vi "data preparer.vi"(2 "error in (no error)":errorcluster, 3 "UI Data":T2) -> (0 "error out":errorcluster, 1 "Prepared (Infix) Data":T1)   [LabVIEW 2020]
uses:
  controls/UI Data.ctl
  <vilib>/Utility/error.llb/Error Cluster From Error Code.vi
  <vilib>/ErrorRing/Error Ring.xnode
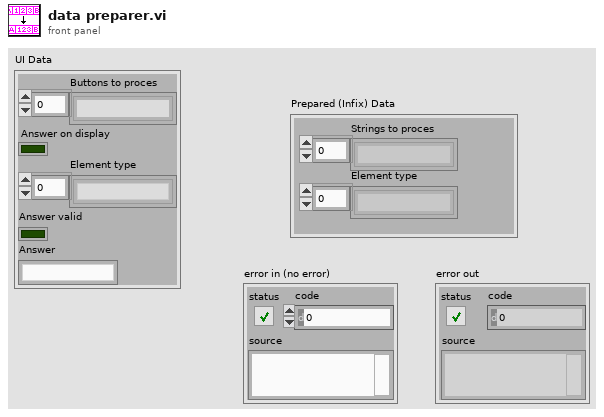
[diagram p1: front panel]
types:
  T1 = cluster{"Strings to proces":string[], "Element type":string[]}
  T2 = typedef "UI Data.ctl" = cluster{"Buttons to proces":string[], "Answer on display":bool, "Element type":string[], "Answer valid":bool, "Answer":string}
  T3 = cluster{"Buttons to proces":string[], "Element type":string[]}
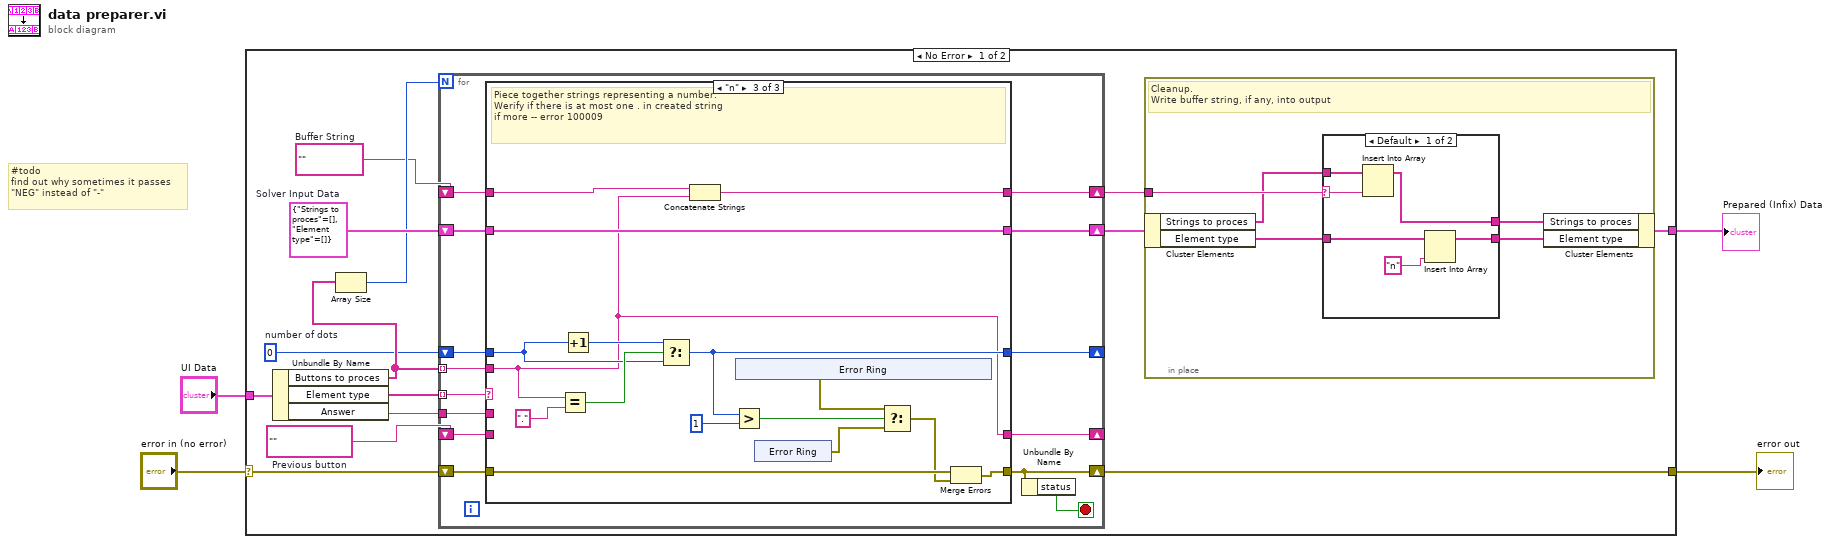
[diagram p0: block diagram]
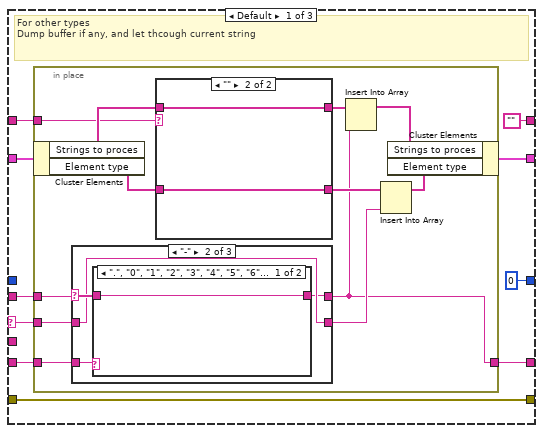
[diagram p3: hidden frame]
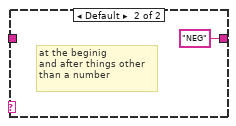
[diagram p5: hidden frame]
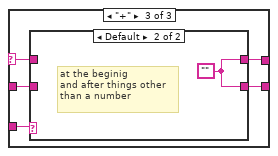
[diagram p6: hidden frame]
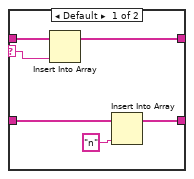
[diagram p8: hidden frame]
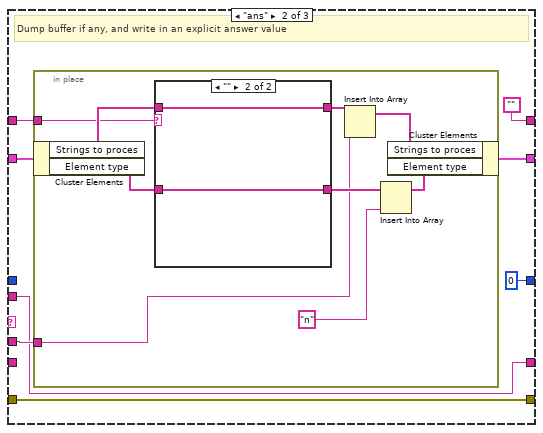
[diagram p9: hidden frame]
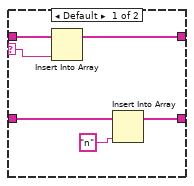
[diagram p10: hidden frame]
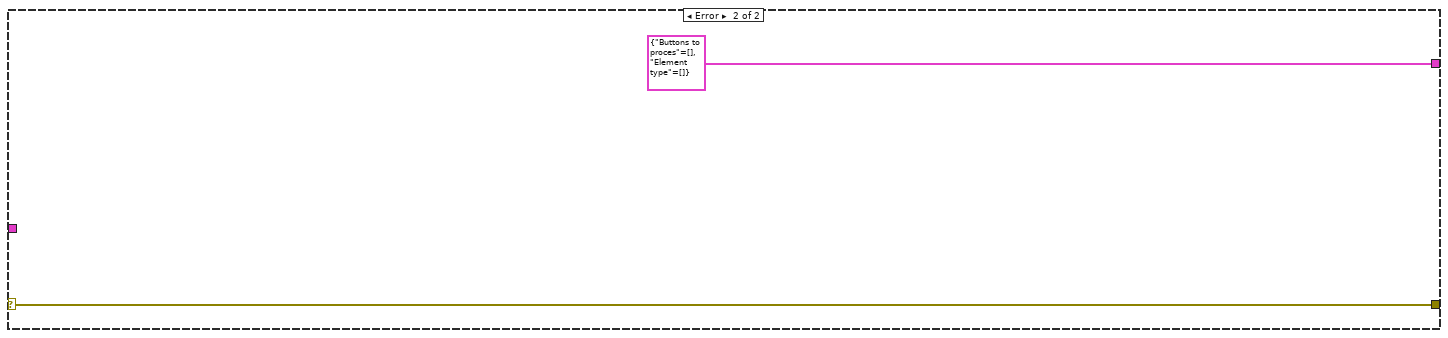
[diagram p11: hidden frame]
diagram:
  # "#todo\nfind out why sometimes it passes\n\"NEG\" instead of \"-\""
  n1 = case shown="No Error" "error in (no error)" {
    selector: "error in (no error)" -> [w16 w140]
    tunnel: [w10 w140] -> w3
    tunnel: "UI Data" -> [w17 _]
    tunnel: [w11 T3 {"Buttons to proces"=[], "Element type"=[]} ("Solver Input Data")] -> w1
    frame No Error {
      w5 = ""  # Previous button
      w6 = 0  # number of dots
      w14 = ""  # Buffer String
      w18 = T1 {"Strings to proces"=[], "Element type"=[]}  # Solver Input Data
      n2 = Unbundle By Name(w17) -> ("Buttons to proces"=w7:string[], "Element type"=w9:string[], "Answer"=w8:string)
      n3 = Array Size(array=w7) -> (size(s)=w15:i32)
      n4 = for {
        N: w15 -> [_]
        shift-right: [w44] -> w12
        shift-left: w18 -> [w45]
        shift-right: [w35] -> w10
        shift-left: w16 -> [w43]
        shift-right: [w41] -> w13
        shift-left: w14 -> [w42]
        tunnel: w7 -> [w40] mode=indexing
        tunnel: w9 -> [w39] mode=indexing
        tunnel: w8 -> [w38]
        shift-right: [w36] -> _
        shift-left: w6 -> [w37]
        shift-right: [w32] -> _
        shift-left: w5 -> [w33]
        stop <- w34 stop-if-true
        n5 = case shown="\"n\"" w39 {
          selector: w39 -> [w52 _ _]
          tunnel: w45 -> [w54 w98 w132]
          tunnel: [w53 w97 w132] -> w44
          tunnel: w43 -> [w55 w99 w131]
          tunnel: [w55 w99 w119] -> w35
          tunnel: w40 -> [w51 w92 w117]
          tunnel: w42 -> [w49 w95 w130]
          tunnel: ["" "" w129] -> w41
          tunnel: w38 -> [_ w94 _]
          tunnel: w37 -> [_ _ w125]
          tunnel: [0 ("number of dots") 0 ("number of dots") w124] -> w36
          tunnel: w33 -> [w47 _ _]
          tunnel: [w46 w92 w117] -> w32
          frame Default {
            # "For other types\nDump buffer if any, and let thcough current string"
            n6 = in-place {
              in-place-border: w52 -> [w60]
              in-place-border: w51 -> [w58]
              in-place-border: w49 -> [w61]
              in-place-border: w47 -> [w57]
              in-place-border: [w56] -> w46
              n7 = in-place-cluster #1(w54) -> ("Strings to proces"=w65:string[], "Element type"=w64:string[])
              n8 = case shown="\"-\"" w58 {
                selector: w58 -> [w68 w71 w79]
                tunnel: [w68 w70 w78] -> w56
                tunnel: w60 -> [w69 w72 w77]
                tunnel: [w69 w72 w76] -> w59
                tunnel: w57 -> [_ w73 w80]
                frame Default {
                  # "things other than \"-\" and \"+\""
                }
                frame "-" {
                  n9 = case shown="\".\", \"0\", \"1\", \"2\", \"3\", \"4\", \"5\", \"6\", \"7\", \"8\", \"9\", \"Ans\"" w73 {
                    tunnel: w71 -> [w74 _]
                    tunnel: [w74 "NEG"] -> w70
                    frame ".", "0", "1", "2", "3", "4", "5", "6", "7", "8", "9", "Ans" {
                    }
                    frame Default {
                      # "at the beginig\nand after things other \nthan a number"
                    }
                  }
                }
                frame "+" {
                  n10 = case shown="Default" w80 {
                    tunnel: w79 -> [w82 _]
                    tunnel: [w82 w83] -> w78
                    tunnel: w77 -> [w81 _]
                    tunnel: [w81 w83] -> w76
                    frame ".", "0", "1", "2", "3", "4", "5", "6", "7", "8", "9" {
                    }
                    frame Default {
                      w83 = ""
                      # "at the beginig\nand after things other \nthan a number"
                    }
                  }
                }
              }
              n11 = case shown="\"\"" w61 {
                selector: w61 -> [w85 _]
                tunnel: w65 -> [w89 w91]
                tunnel: [w88 w91] -> w62
                tunnel: w64 -> [w87 w90]
                tunnel: [w86 w90] -> w63
                frame Default {
                  n12 = Insert Into Array(array=w89, new element=w85) -> (w88:string[])  [unwired: 1 in]
                  n13 = Insert Into Array(array=w87, new element="n" ("new element/subarray")) -> (w86:string[])  [unwired: 1 in]
                }
                frame "" {
                }
              }
              n14 = Insert Into Array(array=w62, new element=w56) -> (w67:string[])  [unwired: 1 in]
              n15 = Insert Into Array(array=w63, new element=w59) -> (w66:string[])  [unwired: 1 in]
              n16 = in-place-cluster #1("Strings to proces"=w67, "Element type"=w66) -> (w53:T1)
            }
          }
          frame "ans" {
            # "Dump buffer if any, and write in an explicit answer value"
            n17 = in-place {
              in-place-border: w95 -> [w102]
              in-place-border: w94 -> [w100]
              n18 = in-place-cluster #2(w98) -> ("Strings to proces"=w106:string[], "Element type"=w105:string[])
              n19 = case shown="\"\"" w102 {
                selector: w102 -> [w110 _]
                tunnel: w106 -> [w114 w116]
                tunnel: [w113 w116] -> w103
                tunnel: w105 -> [w112 w115]
                tunnel: [w111 w115] -> w104
                frame Default {
                  n20 = Insert Into Array(array=w114, new element=w110) -> (w113:string[])  [unwired: 1 in]
                  n21 = Insert Into Array(array=w112, new element="n" ("new element/subarray")) -> (w111:string[])  [unwired: 1 in]
                }
                frame "" {
                }
              }
              n22 = Insert Into Array(array=w103, new element=w100) -> (w108:string[])  [unwired: 1 in]
              n23 = Insert Into Array(array=w104, new element="n") -> (w107:string[])  [unwired: 1 in]
              n24 = in-place-cluster #2("Strings to proces"=w108, "Element type"=w107) -> (w97:T1)
            }
          }
          frame "n" {
            # "Piece together strings representing a number.\nWerify if there is at most one . in created string\nif more -- error 100009"
            n25 = Equal?(x=w117, y=".") -> (x = y?=w127:bool)
            n26 = Increment(x=w125) -> (x+1=w126:i32)
            n27 = Select(t=w126, s=w127, f=w125) -> (s? t:f=w124:i32)
            n28 = Concatenate Strings(w130, w117) -> (w129:string)
            n29 = Greater?(x=w124, y=1) -> (0:w122:bool)
            n30 = xnode "Error Ring"() -> ("error out"=w120:errorcluster)
            n31 = xnode "Error Ring"() -> ("error out"=w121:errorcluster)
            n32 = Select(t=w120, s=w122, f=w121) -> (s? t:f=w118:errorcluster)
            n33 = Merge Errors(w131, w118) -> (w119:errorcluster)
          }
        }
        n34 = Unbundle By Name(w35) -> ("status"=w34:bool)
      }
      n35 = in-place {
        in-place-border: w13 -> [w23]
        # "Cleanup.\nWrite buffer string, if any, into output"
        n36 = in-place-cluster #3(w12) -> ("Strings to proces"=w21:string[], "Element type"=w19:string[])
        n37 = case shown="Default" w23 {
          selector: w23 -> [w25 _]
          tunnel: w21 -> [w29 w30]
          tunnel: [w28 w30] -> w20
          tunnel: w19 -> [w27 w31]
          tunnel: [w26 w31] -> w22
          frame Default {
            n38 = Insert Into Array(array=w29, new element=w25) -> (w28:string[])  [unwired: 1 in]
            n39 = Insert Into Array(array=w27, new element="n" ("new element/subarray")) -> (w26:string[])  [unwired: 1 in]
          }
          frame "" {
          }
        }
        n40 = in-place-cluster #3("Strings to proces"=w20, "Element type"=w22) -> (w11:T1)
      }
    }
    frame Error {
    }
  }
  "Prepared (Infix) Data" <- w1
  "error out" <- w3
